vi "myRIO_BRig_Host_formatData_test1_p2.vi"(7 "input_headers":string[](array[string]), 8 "input_error":errorcluster, 9 "input_Iexist":bool, 10 "input_filePath":path, 11 "input_hdl_Workbooks":refnum<k7>) -> (0 "output_error":errorcluster, 3 "output_hdl_Worksbooks":refnum<k7>)   [LabVIEW 2014]
uses:
  <vilib>/Utility/file.llb/Read From Spreadsheet File (I64).vi
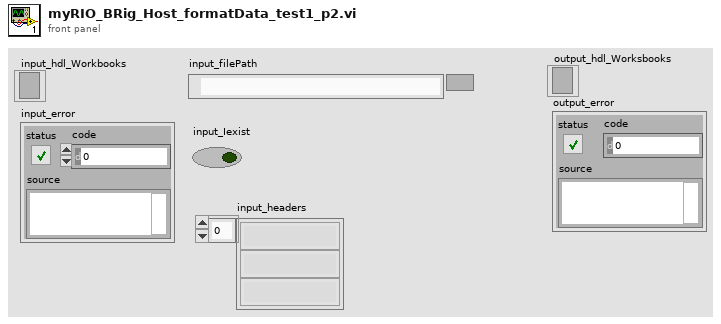
[diagram p1: front panel]
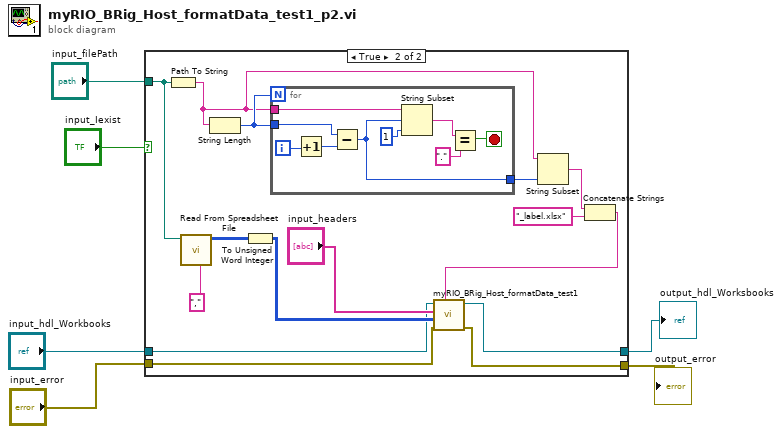
[diagram p0: block diagram]
diagram:
  n1 = case shown="True" "input_Iexist" {
    tunnel: "input_hdl_Workbooks" -> [w8 w13]
    tunnel: "input_error" -> [w7 w12]
    tunnel: [w8 w10] -> w2
    tunnel: [w7 w11] -> w1
    tunnel: "input_filePath" -> [_ w9]
    frame False {
    }
    frame True {
      n2 = Path To String(path=w9) -> (string=w21:string)
      n3 = call-poly <vilib>:"Read From Spreadsheet File.vi"("delimiter (\\t)"="," ("delimiter (\\t)"), "file path (dialog if empty)"=w9) -> ("all rows"=w17:i64[][])  [unwired: 5 in, 4 out]
      n4 = String Length(string=w21) -> (length=w23:i32)
      n5 = To Unsigned Word Integer(number=w17) -> (unsigned 16bit integer=w16:u16[][])
      n6 = for {
        N: w23 -> [_]
        tunnel: w23 -> [w30]
        tunnel: w21 -> [w29]
        tunnel: [w24] -> w22
        i -> [w32]
        stop <- w25 stop-if-true
        n7 = Increment(x=w32) -> (x+1=w31:i32)
        n8 = Subtract(x=w30, y=w31) -> (x-y=w24:i32)
        n9 = String Subset(string=w29, offset (0)=w24, length (rest)=1 ("length (rest)")) -> (substring=w27:string)
        n10 = Equal?(x=w27, y=".") -> (x = y?=w25:bool)
      }
      n11 = String Subset(string=w21, length (rest)=w22) -> (substring=w20:string)  [unwired: 1 in]
      n12 = Concatenate Strings(w20, "_label.xlsx" ("string")) -> (w14:string)
      n13 = call "myRIO_BRig_Host_formatData_test1.vi"("input_filePath"=w14, "input_error"=w12, "input_data"=w16, "input_headers"="input_headers", "input_hdl_Workbooks"=w13) -> ("output_error"=w11:errorcluster, "output_hdl_Worksbooks"=w10:refnum<k7>)  [unwired: 5 in]
    }
  }
  "output_hdl_Worksbooks" <- w2
  "output_error" <- w1
